vi "Copy.vi"(0 "Name Space in":refnum<class "Name Space.lvclass">, 1 "Linked List Ref":refnum<data-value>, 2 "New Parent ID":string, 5 "Test ID":string, 7 "Insertion Index":i32=-1, 9 "Move?":bool, 11 "error in (no error)":errorcluster, 12 "New ID":string, 13 "Data IDs":variant) -> (3 "Linked List Ref out":refnum<data-value>, 6 "Linked List ID out":string, 14 "Data IDs out":variant, 15 "error out":errorcluster)   [LabVIEW 2020, in "Test Executive.lvlib" / "Name Space.lvclass"]
uses:
  <vilib>/gpm_packages/@cs/test-executive/Source/Test Executive/Name Space/Name Space.lvclass
  <vilib>/gpm_packages/@cs/linked-list/Source/Linked List/ILinkedList/ILinked List.lvclass
  <vilib>/gpm_packages/@cs/test-executive/Source/Test Executive/Executioner/Executioner.lvclass
  <vilib>/gpm_packages/@cs/linked-list/Source/Linked List/Linked List Ref/Linked List Ref.lvclass
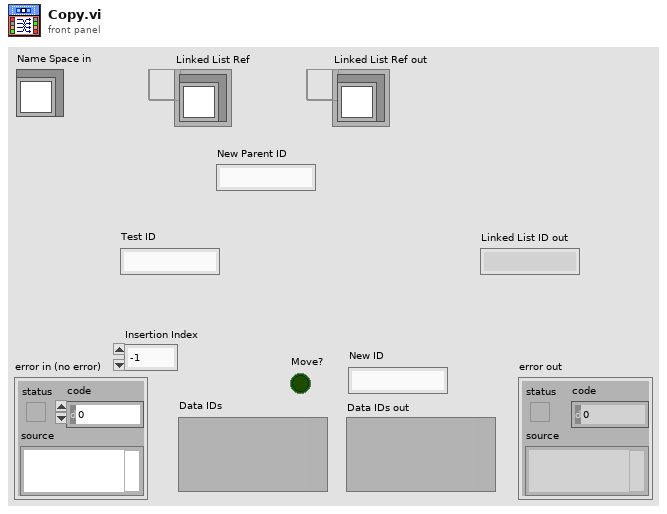
[diagram p1: front panel]
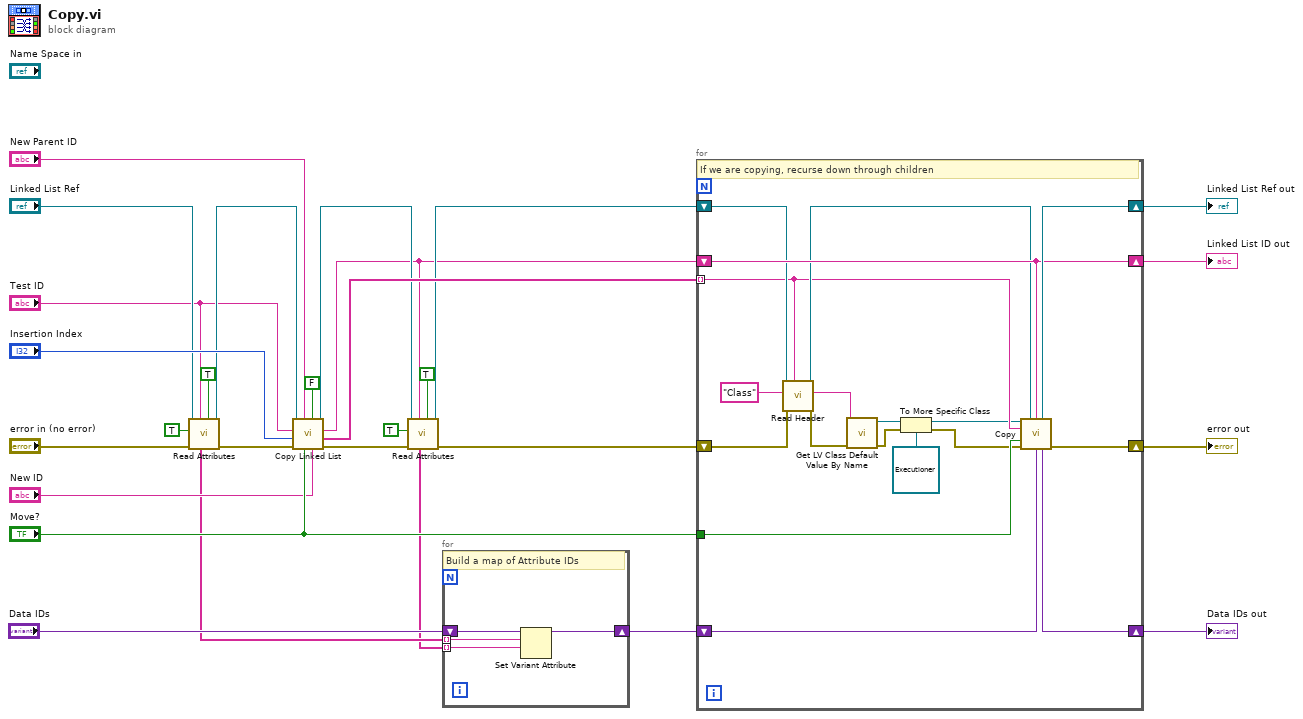
[diagram p0: block diagram]
diagram:
  n1 = call <vilib>:"Read Attributes.vi"("Flatten Pointer?"=TRUE, "Linked List ID"="Test ID", "error in (no error)"="error in (no error)", "Include Private?"=TRUE, "Linked List Ref"="Linked List Ref") -> ("error out"=w8:errorcluster, "Linked List Ref out"=w6:refnum<data-value>, "Data IDs"=w2:string[])  [unwired: 1 in, 3 out]
  n2 = call <vilib>:"Copy Linked List.vi"("New Linked List ID"="New ID", "Recursive? (T)"=FALSE, "Move?"="Move?", "New Parent Linked List ID"="New Parent ID", "error in (no error)"=w8, "Insertion Index"="Insertion Index", "Linked List ID"="Test ID", "Linked List Ref"=w6) -> ("error out"=w17:errorcluster, "Children IDs out"=w27:string[], "Linked List ID out"=w13:string, "Linked List Ref out"=w15:refnum<data-value>)
  n3 = call <vilib>:"Read Attributes.vi"("Flatten Pointer?"=TRUE, "Linked List ID"=w13, "error in (no error)"=w17, "Include Private?"=TRUE, "Linked List Ref"=w15) -> ("error out"=w16:errorcluster, "Linked List Ref out"=w14:refnum<data-value>, "Data IDs"=w1:string[])  [unwired: 1 in, 3 out]
  n4 = for {
    tunnel: w2 -> [w31] mode=indexing
    tunnel: w1 -> [w30] mode=indexing
    shift-right: [w29] -> w4
    shift-left: "Data IDs" -> [w32]
    # "Build a map of Attribute IDs"
    n5 = Set Variant Attribute(Variant=w32, name=w31, value=w30) -> (Variant out=w29:variant)  [unwired: 1 in, 2 out]
  }
  n6 = for {
    shift-right: [w49] -> w26
    shift-left: w14 -> [w38]
    shift-right: [w50] -> w23
    shift-left: w16 -> [w40]
    tunnel: w27 -> [w36] mode=indexing
    tunnel: "Move?" -> [w48]
    shift-right: [w47] -> w20
    shift-left: w13 -> [w47]
    shift-right: [w33] -> w12
    shift-left: w4 -> [w34]
    # "If we are copying, recurse down through children"
    n7 = call <vilib>:"Read Header.vi"("Linked List ID"=w36, "error in (no error)"=w40, "Header Name"="Class", "Linked List Ref"=w38) -> ("error out"=w43:errorcluster, "Header Value"=w45:string, "Linked List Ref out"=w37:refnum<data-value>)  [unwired: 4 in, 1 out]
    n8 = call <vilib>:"Get LV Class Default Value By Name.vi"("error in (no error)"=w43, "class name"=w45) -> ("error out"=w42:errorcluster, "object"=w44:refnum<class>)  [unwired: 8 in]
    n9 = To More Specific Class(target class=refnum<class "Executioner.lvclass"> refnum ("Test Executive.lvlib:Executioner.lvclass"), reference=w44, error in=w42) -> (specific class reference=w35:refnum<class "Executioner.lvclass">, error out=w39:errorcluster)
    n10 = call-dynamic "Copy.vi"("Executioner in"=w35, "Linked List Ref"=w37, "New Parent ID"=w47, "Test ID"=w36, "Move?"=w48, "error in (no error)"=w39, "Data IDs"=w34) -> ("Linked List Ref out"=w49:refnum<data-value>, "Data IDs out"=w33:variant, "error out"=w50:errorcluster)  [unwired: 5 in, 1 out]
  }
  "error out" <- w23
  "Linked List Ref out" <- w26
  "Linked List ID out" <- w20
  "Data IDs out" <- w12
